vi "卡尔曼滤波.vi"(5 "R":dbl, 7 "Q":dbl, 8 "上一轮估算协方差":dbl, 10 "输入":dbl, 11 "上一轮输出":dbl) -> (0 "本轮估算协方差":dbl, 3 "本轮输出":dbl)   [LabVIEW 2020]
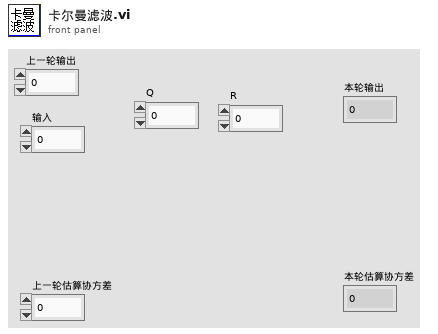
[diagram p1: front panel]
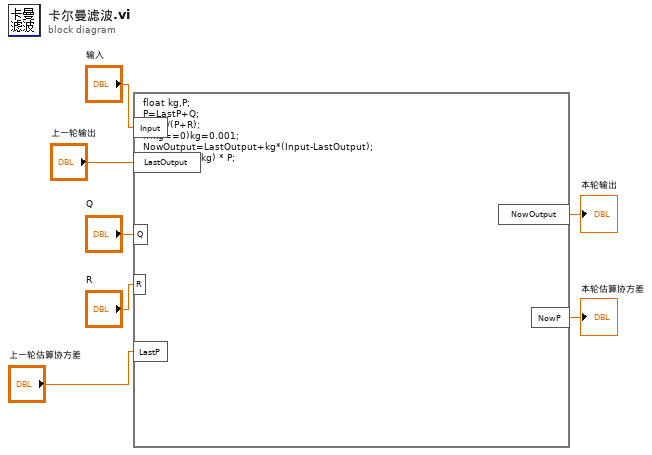
[diagram p0: block diagram]
diagram:
  n1 = formula code="float kg,P;\nP=LastP+Q;\nkg=P/(P+R);\nif(kg==0)kg=0.001;\nNowOutput=LastOutput+kg*(Input-LastOutput);\nNowP = (1 - kg) * P;"("Input"="输入", "LastOutput"="上一轮输出", "Q"="Q", "R"="R", "LastP"="上一轮估算协方差") -> ("NowOutput"=→"本轮输出":dbl, "NowP"=→"本轮估算协方差":dbl)
